vi "receiveDecodeAndDoKalman.vi"(0 "Vision in":refnum<class "Vision.lvclass">, 1 "NewCameras":T4[](array[typedef]) {"robots_blue"."height" format="%+4.3f"; "robots_blue"."pixel_y" format="%+4.3f"; "robots_blue"."pixel_x" format="%+4.3f"; "robots_blue"."orientation" format="%+4.3f"; "robots_blue"."y" format="%+4.3f"; "robots_blue"."confidence" format="%4.3f"; "robots_blue"."x" format="%+4.3f"; "robots_yellow"."height" format="%+4.3f"; "robots_yellow"."pixel_y" format="%+4.3f"; "robots_yellow"."pixel_x" format="%+4.3f"; "robots_yellow"."orientation" format="%+4.3f"; "robots_yellow"."y" format="%+4.3f"; "robots_yellow"."confidence" format="%4.3f"; "robots_yellow"."x" format="%+4.3f"}, 3 "Field Size":T6, 4 "Estimador":T8=enum."Nenhum", 5 "error in (no error)":errorcluster, 6 "cameras array":dbl[](array[numeric]), 7 "team/side":u16[](array[numeric]), 8 "timeToValidateBall":dbl=0.5, 10 "Com UDP":T3={"UDP GrSim TX"=TRUE, "Address:"="192.168.1.46", "Port:"=20011}, 11 "BallOut":bool, 12 "Life Time":dbl=4.0, 18 "max ball vel":dbl) -> (14 "Vision out":refnum<class "Vision.lvclass">, 15 "Frame and Field Size out":T7 {"Detection Frame Out"."robots_blue"."height" format="%+4.3f"; "Detection Frame Out"."robots_blue"."pixel_y" format="%+4.3f"; "Detection Frame Out"."robots_blue"."pixel_x" format="%+4.3f"; "Detection Frame Out"."robots_blue"."orientation" format="%+4.3f"; "Detection Frame Out"."robots_blue"."y" format="%+4.3f"; "Detection Frame Out"."robots_blue"."confidence" format="%4.3f"; "Detection Frame Out"."robots_blue"."x" format="%+4.3f"; "Detection Frame Out"."robots_yellow"."height" format="%+4.3f"; "Detection Frame Out"."robots_yellow"."pixel_y" format="%+4.3f"; "Detection Frame Out"."robots_yellow"."pixel_x" format="%+4.3f"; "Detection Frame Out"."robots_yellow"."orientation" format="%+4.3f"; "Detection Frame Out"."robots_yellow"."y" format="%+4.3f"; "Detection Frame Out"."robots_yellow"."confidence" format="%4.3f"; "Detection Frame Out"."robots_yellow"."x" format="%+4.3f"}, 19 "error out":errorcluster)   [LabVIEW 2020, in "Vision.lvclass"]
uses:
  Vision.lvclass
  Old vision/Controls/Estimadores.ctl
  Old vision/Controls/SSL Field State.ctl
  Old vision/Controls/SSL Detection Frame.ctl
  Old vision/Controls/SSL Detection Robot.ctl
  <vilib>/Analysis/Matrix/Datatypes/RealMatrix.ctl
  Old vision/Controls/SSL Detection Ball.ctl
  Controls/ComUDP.ctl
  <vilib>/Analysis/Matrix/NI_Matrix.lvlib
panel:
  in  "empty_balls":T1[](array[typedef])
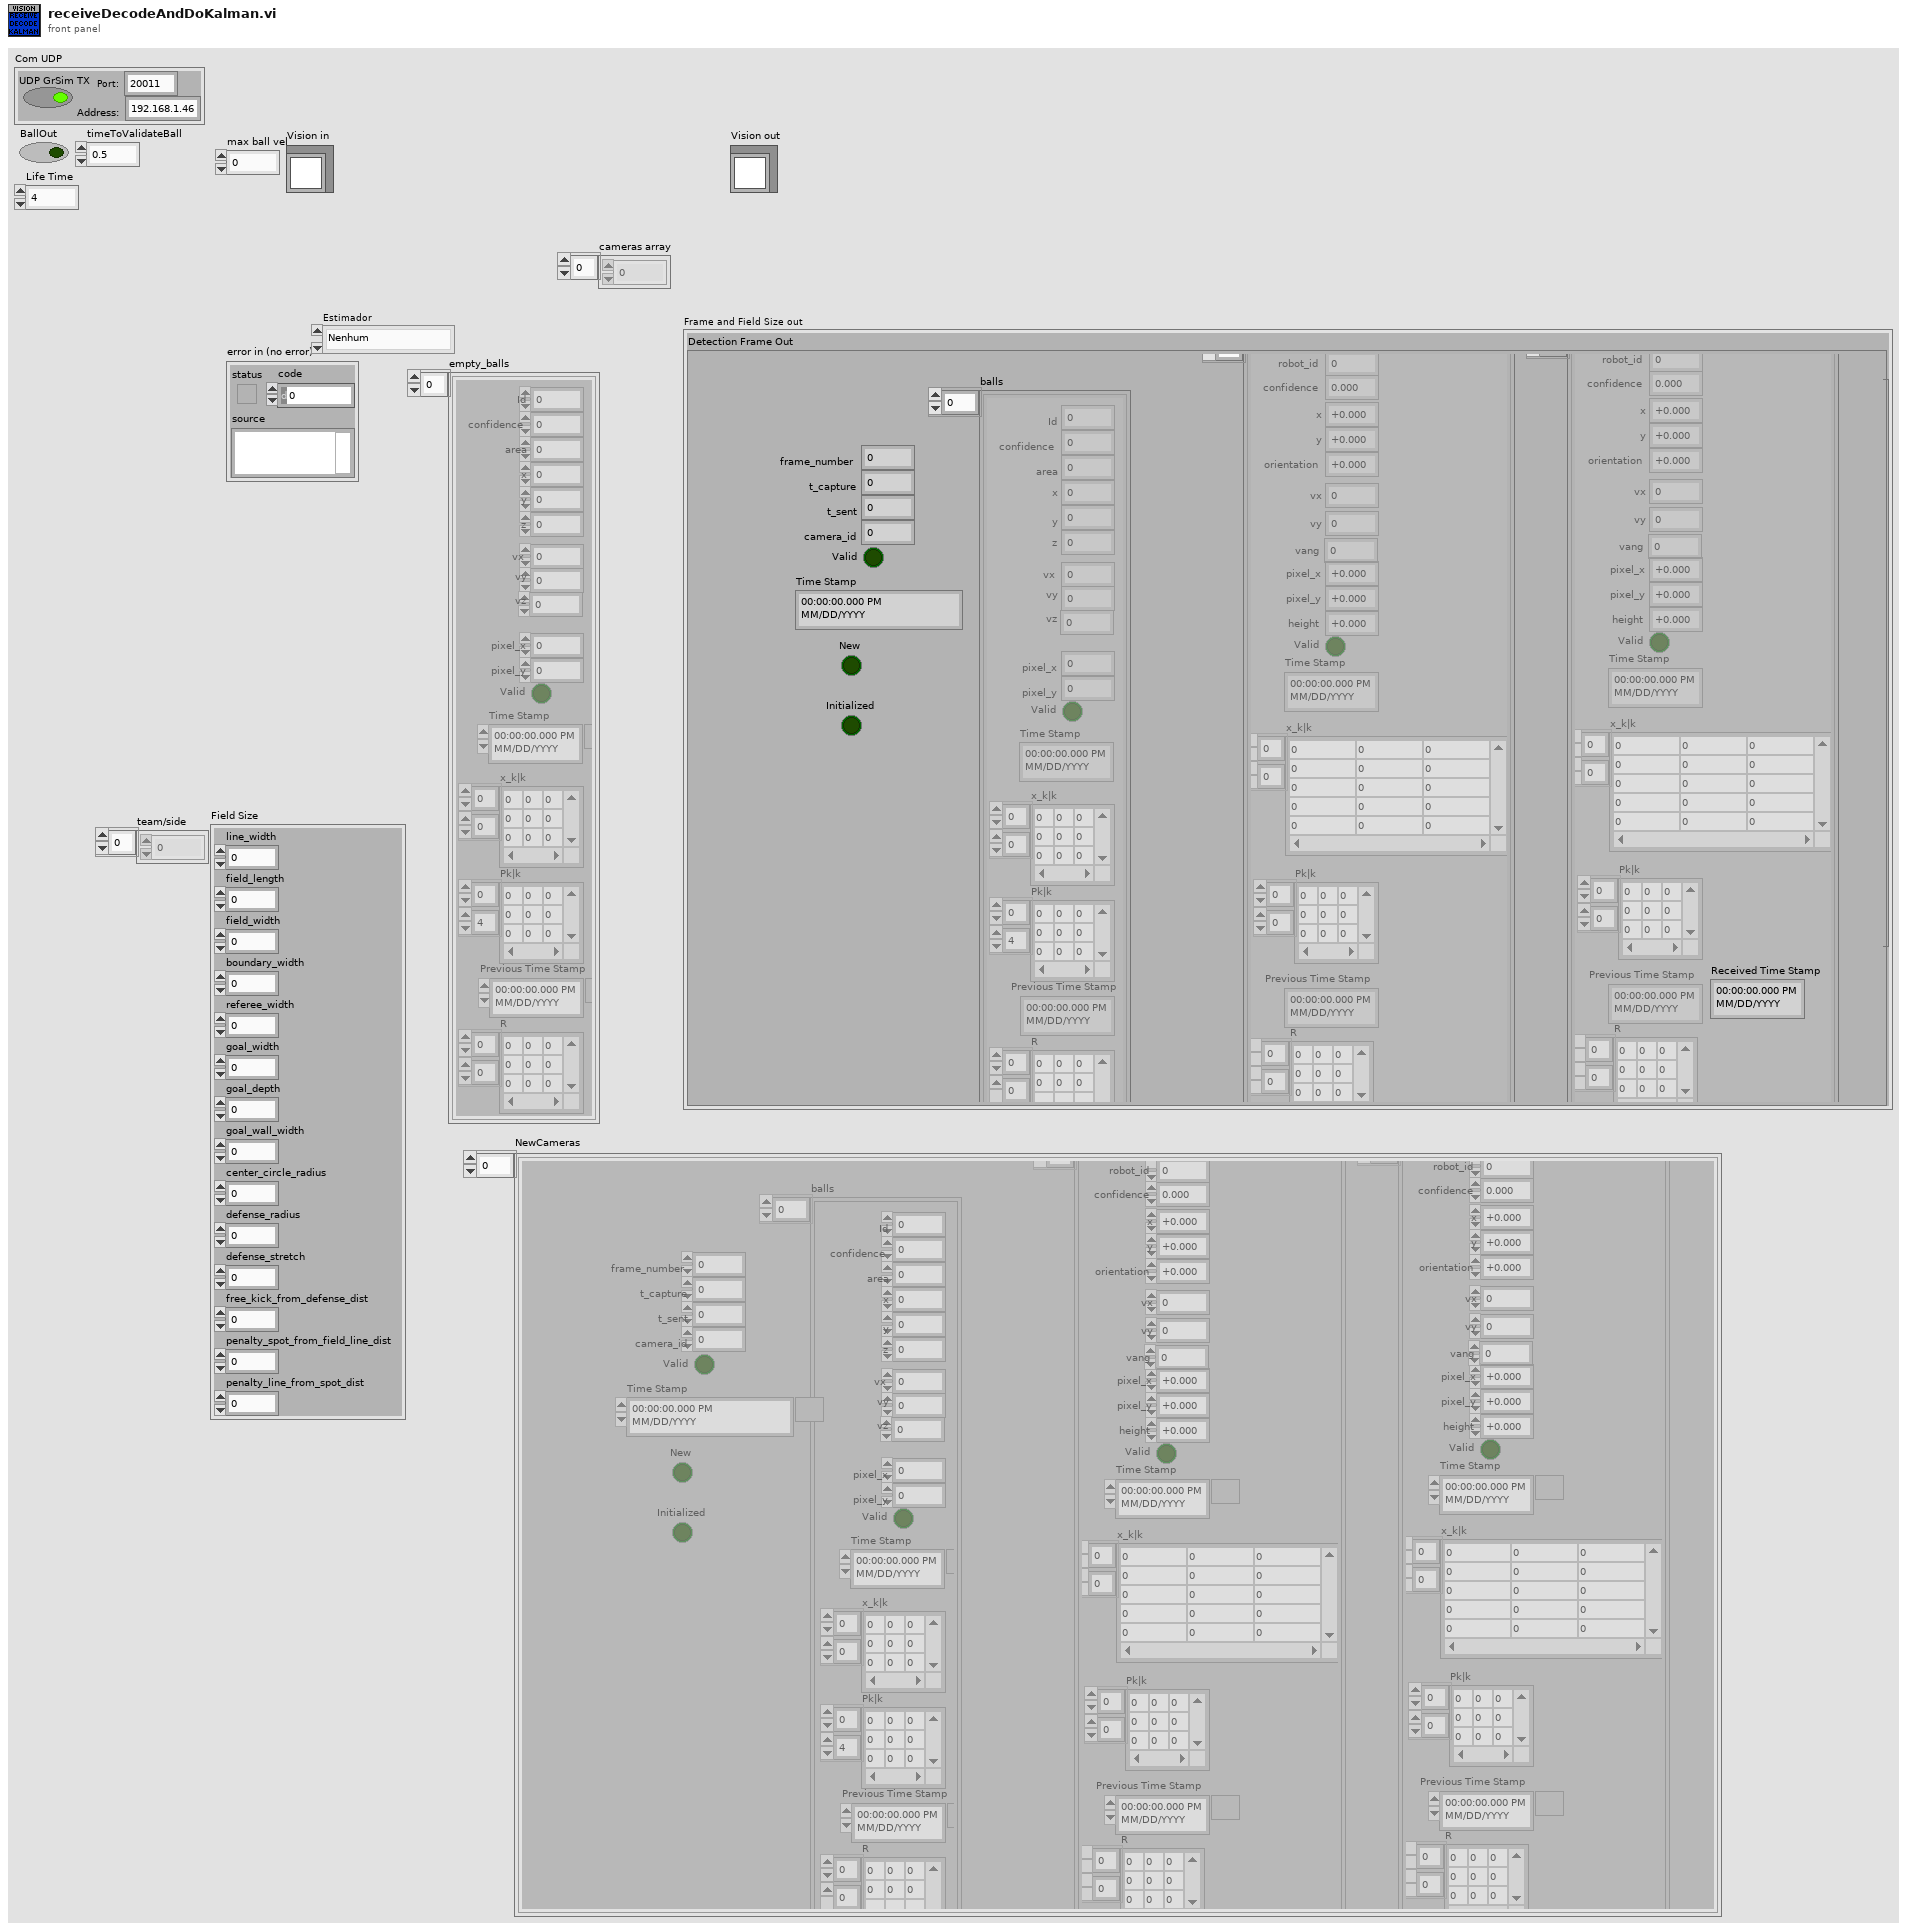
[diagram p1: front panel]
types:
  T1 = typedef "SSL Detection Ball.ctl" = cluster{"x":sgl, "area":u32, "confidence":sgl, "y":sgl, "z":sgl, "pixel_x":sgl, "pixel_y":sgl, "Valid":bool, "Time Stamp":timestamp, "x_k|k":T2, "Pk|k":T2, "Id":u32, "Previous Time Stamp":timestamp, "R":T2, " vx":sgl, "vy":dbl, "vz":dbl}
  T2 = typedef "NI_Matrix.lvlib/RealMatrix.ctl" = dbl[][]
  T3 = typedef "ComUDP.ctl" = cluster{"UDP GrSim TX":bool, "Address:":string, "Port:":u16}
  T4 = typedef "SSL Detection Frame.ctl" = cluster{"frame_number":u32, "t_capture":dbl, "t_sent":dbl, "camera_id":u32, "robots_yellow":T5[], "robots_blue":T5[], "balls":T1[], "Valid":bool, "Time Stamp":timestamp, "New":bool, "Initialized":bool}
  T5 = typedef "SSL Detection Robot.ctl" = cluster{"x":sgl, "robot_id":u32, "confidence":sgl, "y":sgl, "orientation":sgl, "pixel_x":sgl, "pixel_y":sgl, "height":sgl, "Valid":bool, "Time Stamp":timestamp, "x_k|k":T2, "Pk|k":T2, "Previous Time Stamp":timestamp, "R":T2, "vx":dbl, "vy":dbl, "vang":dbl}
  T6 = cluster{"line_width":u32, "field_length":u32, "field_width":u32, "boundary_width":u32, "referee_width":u32, "goal_width":u32, "goal_depth":u32, "goal_wall_width":u32, "center_circle_radius":u32, "defense_radius":u32, "defense_stretch":u32, "free_kick_from_defense_dist":u32, "penalty_spot_from_field_line_dist":u32, "penalty_line_from_spot_dist":u32}
  T7 = typedef "SSL Field State.ctl" = cluster{"Detection Frame Out":T4, "Field Size Out":cluster{"line_width":u32, "field_length":u32, "field_width":u32, "boundary_width":u32, "referee_width":u32, "goal_width":u32, "goal_depth":u32, "goal_wall_width":u32, "center_circle_radius":u32, "defense_radius":u32, "defense_stretch":u32, "free_kick_from_defense_dist":u32, "penalty_spot_from_field_line_dist":u32, "penalty_line_from_spot_dist":u32}, "Received Time Stamp":timestamp}
  T8 = typedef "Estimadores.ctl" = enum16{"Variable2ndDerivate", "4thDerivate", "2ndDerivate", "Nenhum", "Simples", "Kalman"}
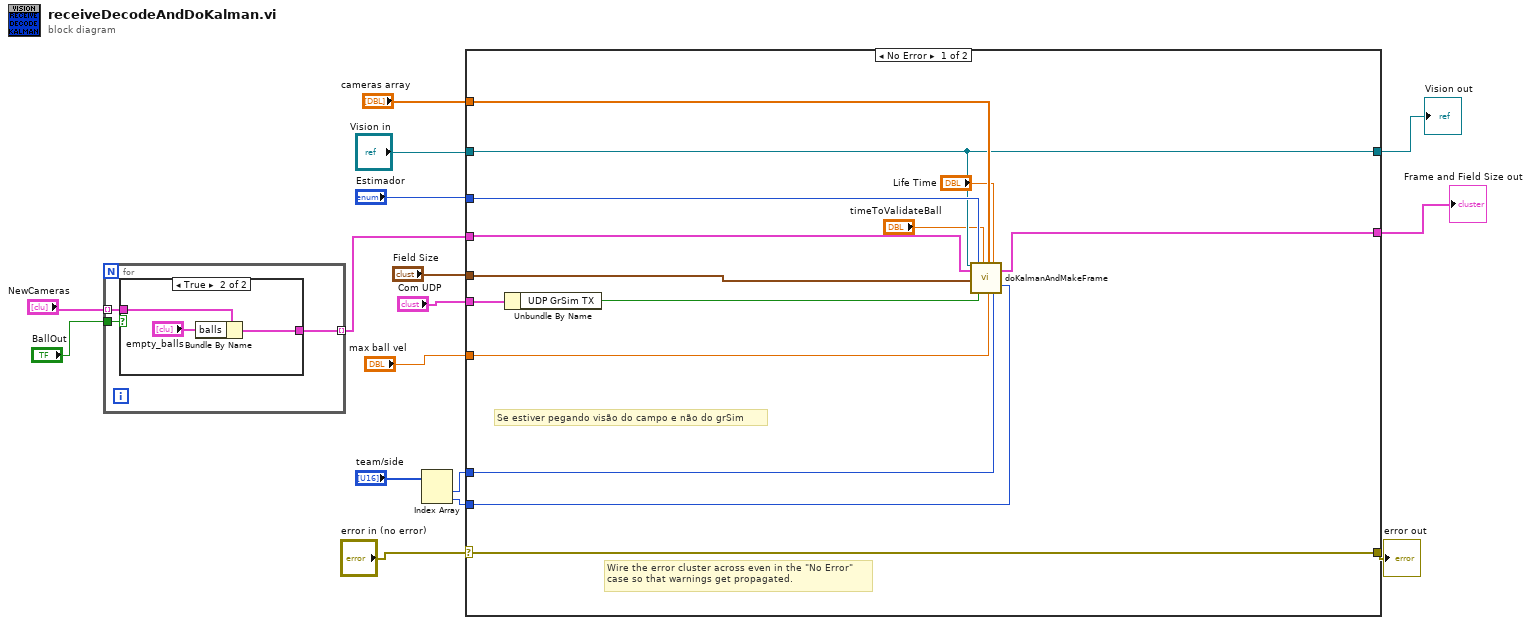
[diagram p0: block diagram]
diagram:
  n1 = for {
    tunnel: "NewCameras" -> [w19] mode=indexing
    tunnel: [w18] -> w2 mode=indexing
    tunnel: "BallOut" -> [w17]
    n2 = case shown="True" w17 {
      tunnel: w19 -> [w20 w23]
      tunnel: [w20 w21] -> w18
      frame False {
      }
      frame True {
        n3 = Bundle By Name(cluster=w23, "balls"="empty_balls") -> (w21:T4)
      }
    }
  }
  n4 = Index Array(array="team/side") -> (element #1=w10:u16, element #2=w9:u16)  [unwired: 2 in]
  n5 = case shown="No Error" "error in (no error)" {
    selector: "error in (no error)" -> [w37 w39]
    tunnel: [w37 w39] -> w15
    tunnel: [w30 w38] -> w13
    tunnel: "Vision in" -> [w30 w38]
    tunnel: [w36 _] -> w12
    tunnel: w10 -> [w35 _]
    tunnel: w9 -> [w34 _]
    tunnel: "Estimador" -> [w33 _]
    tunnel: "cameras array" -> [w32 _]
    tunnel: "max ball vel" -> [w31 _]
    tunnel: "Field Size" -> [w29 _]
    tunnel: w2 -> [w26 _]
    tunnel: "Com UDP" -> [w28 _]
    frame No Error {
      # "Se estiver pegando visão do campo e não do grSim"
      # "Wire the error cluster across even in the \"No Error\"\ncase so that warnings get propagated."
      n6 = Unbundle By Name(w28) -> ("UDP GrSim TX"=w27:bool)
      n7 = call "doKalmanAndMakeFrame.vi"("Vision in"=w30, "NewCameras"=w26, "Field Size"=w29, "Estimador"=w33, "grSim"=w27, "timeToValidateBall"="timeToValidateBall", "cameras array"=w32, "max ball vel"=w31, "Life Time"="Life Time", "Team"=w35, "Side"=w34) -> ("Frame and Field Size out"=w36:T7)  [unwired: 6 in, 2 out]
    }
    frame Error {
    }
  }
  "error out" <- w15
  "Vision out" <- w13
  "Frame and Field Size out" <- w12
